vi "MHM Save Register Ex.vi"(6 "pulData":u32[](array[numeric]), 7 "pulNumberOfBytes":u32, 8 "error in (no error)":errorcluster, 9 "ulAdr":u32, 10 "pcFilename":string, 11 "ulMHMHandle":u32) -> (0 "error out (no error)":errorcluster, 2 "pulNumberOfBytes out":u32, 3 "function return":u32)   [LabVIEW 2017, in "MHM_1SL_interface.lvlib"]
uses:
  MHM_1SL_interface.lvlib
  SSI_Tool/DUT_Interface/lv_interface/lib/MHM_1SL_interface.dll
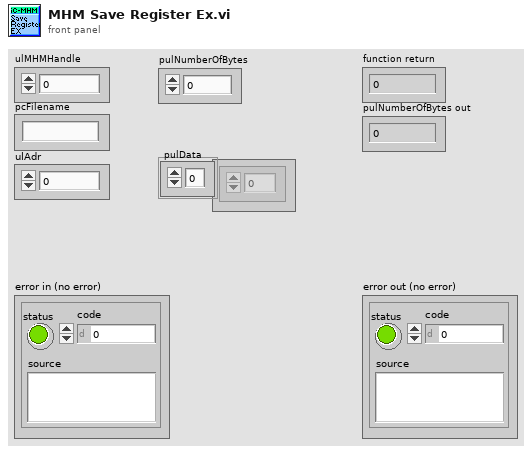
[diagram p1: front panel]
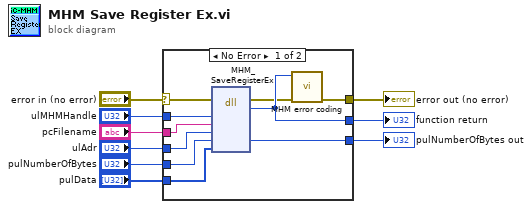
[diagram p0: block diagram]
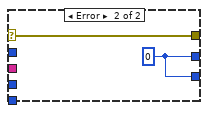
[diagram p2: hidden frame]
diagram:
  n1 = case shown="No Error" "error in (no error)" {
    selector: "error in (no error)" -> [w10 w21]
    tunnel: [w19 w20] -> w9
    tunnel: "ulMHMHandle" -> [w18 _]
    tunnel: "pcFilename" -> [w17 _]
    tunnel: "ulAdr" -> [w16 _]
    tunnel: "pulNumberOfBytes" -> [w15 _]
    tunnel: [w14 w20] -> w4
    tunnel: [w12 w21] -> w3
    tunnel: "pulData" -> [w11 _]
    frame No Error {
      n2 = dll-call lib="C:/workspace/project/scancon/sw/SSI_Tool/DUT_Interface/lv_interface/lib/MHM_1SL_interface.dll" fn="MHM_SaveRegisterEx"(error in=w10, "ulMHMHandle"=w18, "pcFilename"=w17, "ulAdr"=w16, "ulNumberOfBytes"=w15, "pulData"=w11) -> (error out=w13:errorcluster, "return type"=w19:u32, "ulNumberOfBytes"=w14:u32)  [unwired: 6 in, 1 out]
      n3 = call "MHM error coding.vi"("error in (no error)"=w13, "function return in"=w19) -> ("error out"=w12:errorcluster)  [unwired: 9 in]
    }
    frame Error {
      w20 = u32 0 ("return type")
    }
  }
  "function return" <- w9
  "pulNumberOfBytes out" <- w4
  "error out (no error)" <- w3
